vi "save channels to separate multi-tiff files.vi"(8 "frame number in":i32, 9 "last frame":bool, 11 "image data in":dbl[][](array[numeric])) -> ()   [LabVIEW 2012]
doc: "SciScan 1.2 160622"
uses:
  Custom Controls/file format type def.ctl
  GFG/GFGpathGet.vi
  GFG/GFGnumericGet.vi
  GFG/GFGstringGet.vi
  Libtiff3/libtiff3.llb/libtiff3.lvlib
  GFG/GFG library.lvlib
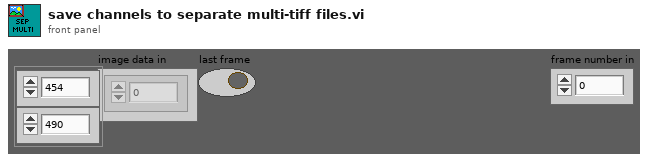
[diagram p1: front panel]
types:
  T1 = typedef "file format type def.ctl" = enum16{"16bit raw", "32bit raw", "16bit multi-tiff (interleave)", "16bit multi-tiff (separate)", "16bit multi-tiff (stacked)", "32bit multi-tiff (interleave)", "32bit multi-tiff (separate)", "32bit multi-tiff (stacked)", "16bit tiff series (interleave)", "16bit tiff series (separate)", "16bit tiff series (stacked)", "32bit tiff series (interleave)", "32bit tiff series (separate)", "32bit tiff series (stacked)"}
  T2 = cluster{"no..of.frames.to.acquire":dbl, "x.pixels":dbl, "y.pixels":dbl, "x.pixel.sz":dbl, "y.pixel.sz":dbl}
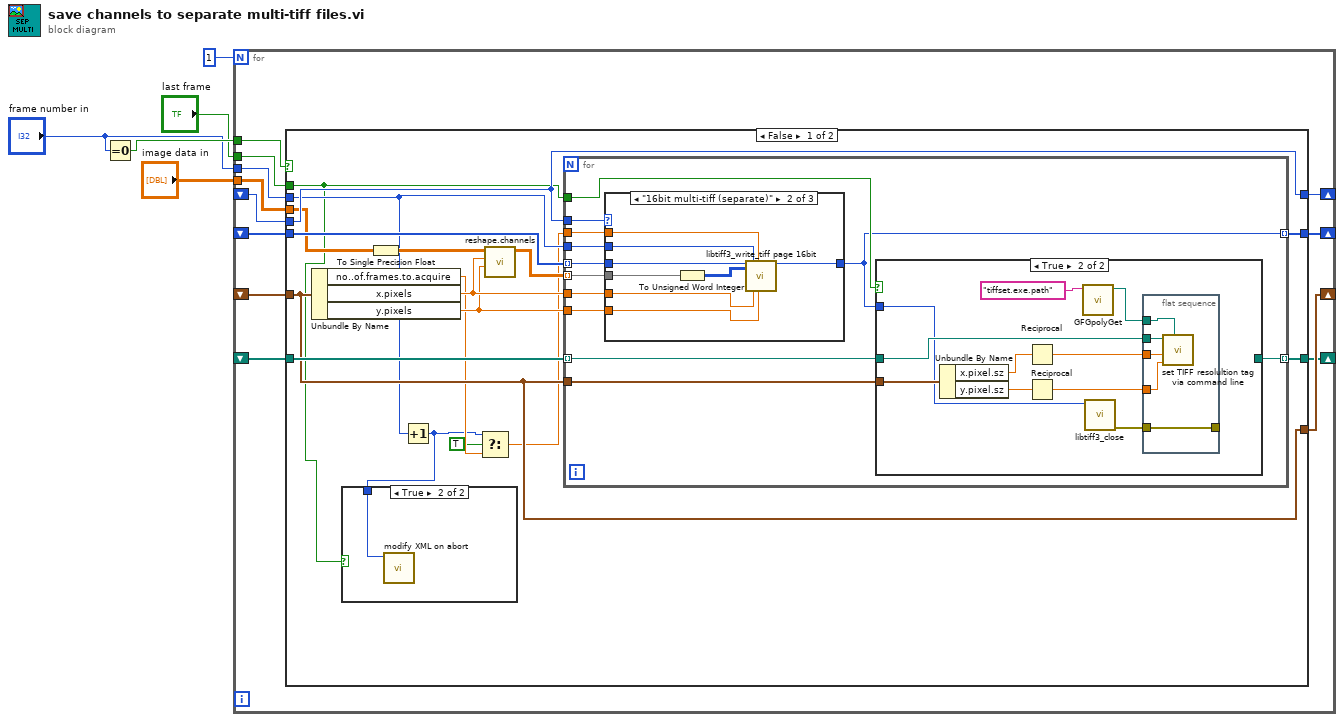
[diagram p0: block diagram]
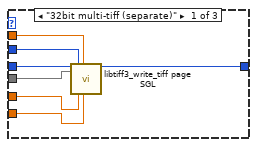
[diagram p3: hidden frame]
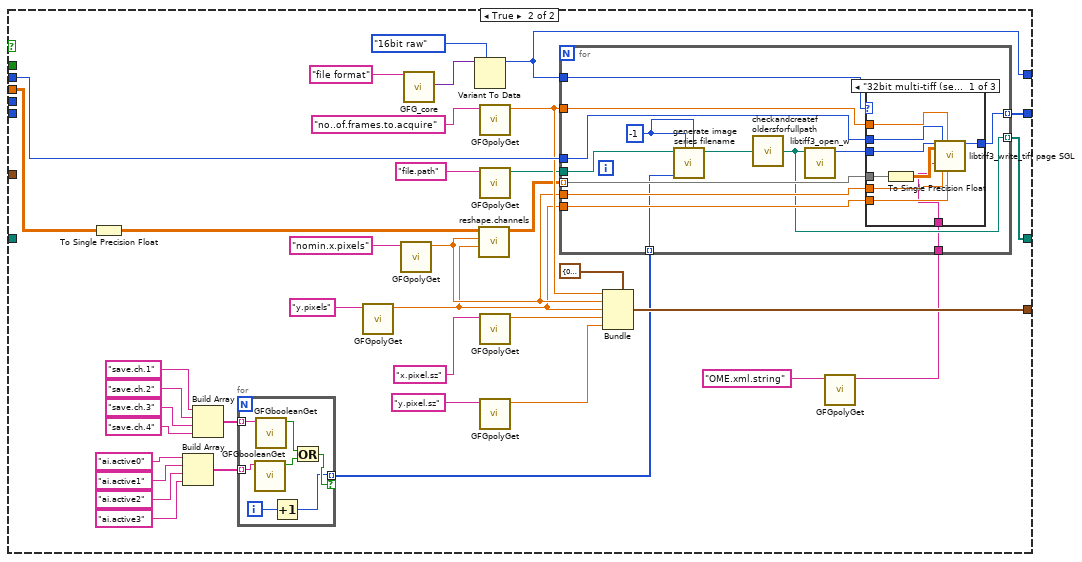
[diagram p6: hidden frame]
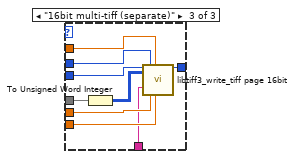
[diagram p8: hidden frame]
diagram:
  n1 = Equal To 0?(x="frame number in") -> (x = 0?=w4:bool)
  n2 = for {
    N: 1 -> [_]
    tunnel: w4 -> [w17]
    shift-right: [w16] -> _
    shift-left: _ -> [w15]
    tunnel: "image data in" -> [w14]
    shift-right: [w13] -> _
    shift-left: _ -> [w12]
    shift-right: [w11] -> _
    shift-left: _ -> [w10]
    shift-right: [w9] -> _
    shift-left: _ -> [w8]
    tunnel: "last frame" -> [w7]
    tunnel: "frame number in" -> [w6]
    n3 = case shown="False" w17 {
      tunnel: w12 -> [w31 _]
      tunnel: [w29 w100] -> w16
      tunnel: w15 -> [w33 _]
      tunnel: w14 -> [w28 w96]
      tunnel: [w31 w103] -> w13
      tunnel: [w30 w104] -> w11
      tunnel: w10 -> [w30 _]
      tunnel: [w32 w93] -> w9
      tunnel: w8 -> [w34 _]
      tunnel: w7 -> [w20 _]
      tunnel: w6 -> [w23 w102]
      frame False {
        n4 = Unbundle By Name(w30) -> ("no..of.frames.to.acquire"=w22:dbl, "x.pixels"=w25:dbl, "y.pixels"=w24:dbl)
        n5 = To Single Precision Float(number=w28) -> (single precision float=w27:sgl[][])
        n6 = Increment(x=w23) -> (x+1=w19:i32)
        n7 = case shown="True" w20 {
          tunnel: w19 -> [_ w35]
          frame False {
          }
          frame True {
            n8 = call "modify XML on abort.vi"("frame number"=w35) -> ()  [unwired: 10 in, 1 out]
          }
        }
        n9 = Select(t=w19, s=TRUE, f=w22) -> (s? t:f=w21:dbl)
        n10 = call "reshape.channels.vi"("y.pixels"=w24, "x.pixels"=w25, "element"=w27) -> ("Array"=w26:dbl[][][])  [unwired: 8 in]
        n11 = for {
          tunnel: w20 -> [w47]
          tunnel: w34 -> [w46] mode=indexing
          tunnel: w26 -> [w45] mode=indexing
          tunnel: w33 -> [w44] mode=indexing
          tunnel: [w43] -> w32 mode=indexing
          tunnel: w21 -> [w42]
          tunnel: w23 -> [w41]
          tunnel: w25 -> [w40]
          tunnel: w24 -> [w39]
          tunnel: w31 -> [w38]
          tunnel: w30 -> [w37]
          tunnel: [w36] -> w29 mode=indexing
          n12 = case shown="\"16bit multi-tiff (separate)\"" w38 {
            tunnel: w45 -> [w48 w62 _]
            tunnel: w44 -> [w54 w60 w63]
            tunnel: [w51 w59 w63] -> w36
            tunnel: w42 -> [w52 w58 _]
            tunnel: w41 -> [w53 w57 _]
            tunnel: w40 -> [w50 w56 _]
            tunnel: w39 -> [w49 w55 _]
            frame "32bit multi-tiff (separate)" {
              n13 = call "libtiff3_write_tiff page SGL.vi"("Handle"=w54, "Image Pixels (Float)"=w48, "page"=w53, "x.pixels"=w50, "totalpages"=w52, "y.pixels"=w49) -> ("Handle out"=w51:i32)  [unwired: 12 in, 1 out]
            }
            frame "16bit multi-tiff (separate)" {
              n14 = To Unsigned Word Integer(number=w62) -> (unsigned 16bit integer=w61:u16[][])
              n15 = call "libtiff3_write_tiff page 16bit.vi"("Handle"=w60, "Image Pixels (U16)"=w61, "page"=w57, "x.pixels"=w56, "totalpages"=w58, "y.pixels"=w55) -> ("Handle out"=w59:i32)  [unwired: 12 in, 1 out]
            }
            frame Default {
            }
          }
          n16 = case shown="True" w47 {
            tunnel: w37 -> [_ w69]
            tunnel: w46 -> [w64 w68]
            tunnel: w36 -> [_ w67]
            tunnel: [w64 _] -> w43
            frame False {
            }
            frame True {
              n17 = Unbundle By Name(w69) -> ("x.pixel.sz"=w70:dbl, "y.pixel.sz"=w71:dbl)
              n18 = Reciprocal(x=w70) -> (1/x=w72:dbl)
              n19 = Reciprocal(x=w71) -> (1/x=w73:dbl)
              n20 = call-poly "GFGpolyGet.vi"("Variable Name in"="tiffset.exe.path") -> ("Path"=w65:path)  [unwired: 8 in, 2 out]
              n21 = call "libtiff3_close.vi"("Handle"=w67) -> ("error out"=w74:errorcluster)  [unwired: 9 in]
              n22 = flat-sequence {
                tunnel: w68 -> [w79]
                tunnel: w74 -> [w76]
                tunnel: w72 -> [w78]
                tunnel: w73 -> [w77]
                tunnel: [w76] -> _
                tunnel: w65 -> [w75]
                frame #0 {
                  n23 = call "set TIFF resolultion tag via command line.vi"("tiffset.exe file path"=w75, "y pixels per m"=w77, "x pixels per m"=w78, "TIFF file path"=w79) -> ()  [unwired: 8 in]
                }
              }
            }
          }
        }
      }
      frame True {
        n24 = To Single Precision Float(number=w96) -> (single precision float=w99:sgl[][])
        n25 = Build Array("ai.active0" ("Variable Name in"), "ai.active1" ("Variable Name in"), "ai.active2" ("Variable Name in"), "ai.active3" ("Variable Name in")) -> (w82:string[])
        n26 = Build Array("save.ch.1" ("Variable Name in"), "save.ch.2" ("Variable Name in"), "save.ch.3" ("Variable Name in"), "save.ch.4" ("Variable Name in")) -> (w87:string[])
        n27 = for {
          tunnel: w87 -> [w123] mode=indexing
          tunnel: w82 -> [w122] mode=indexing
          tunnel: [w117] -> w81 mode=indexing if=w118
          i -> [w119]
          n28 = call "GFGbooleanGet.vi"("Variable Name in"=w122) -> ("Boolean Value OUT"=w121:bool)  [unwired: 9 in, 1 out]
          n29 = call "GFGbooleanGet.vi"("Variable Name in"=w123) -> ("Boolean Value OUT"=w120:bool)  [unwired: 9 in, 1 out]
          n30 = Increment(x=w119) -> (x+1=w117:i32)
          n31 = Or(x=w120, y=w121) -> (x .or. y?=w118:bool)
        }
        n32 = call-poly "GFGpolyGet.vi"("Variable Name in"="y.pixels" ("Tag in")) -> ("Numeric"=w97:dbl)  [unwired: 8 in, 2 out]
        n33 = call-poly "GFGpolyGet.vi"("Variable Name in"="nomin.x.pixels" ("Tag in")) -> ("Numeric"=w98:dbl)  [unwired: 8 in, 2 out]
        n34 = call "GFG_core.vi"("Variable Name in"="file format") -> ("Variant Out"=w115:variant)  [unwired: 12 in, 6 out]
        n35 = Variant To Data(type=file_format_type_def."16bit raw" ("file format"), Variant=w115) -> (data=w103:T1)  [unwired: 1 in, 1 out]
        n36 = call "reshape.channels.vi"("y.pixels"=w97, "x.pixels"=w98, "element"=w99) -> ("Array"=w95:dbl[][][])  [unwired: 8 in]
        n37 = call-poly "GFGpolyGet.vi"("Variable Name in"="no..of.frames.to.acquire") -> ("Numeric"=w101:dbl)  [unwired: 8 in, 2 out]
        n38 = call-poly "GFGpolyGet.vi"("Variable Name in"="file.path") -> ("Path"=w94:path)  [unwired: 8 in, 2 out]
        n39 = call-poly "GFGpolyGet.vi"("Variable Name in"="x.pixel.sz" ("Tag in")) -> ("Numeric"=w107:dbl)  [unwired: 8 in, 2 out]
        n40 = call-poly "GFGpolyGet.vi"("Variable Name in"="y.pixel.sz" ("Tag in")) -> ("Numeric"=w106:dbl)  [unwired: 8 in, 2 out]
        n41 = Bundle(cluster=T2 {"no..of.frames.to.acquire"=0.0, "x.pixels"=0.0, "y.pixels"=0.0, "x.pixel.sz"=0.0, "y.pixel.sz"=0.0} ("output cluster"), "no..of.frames.to.acquire"=w101, "x.pixels"=w98, "y.pixels"=w97, "x.pixel.sz"=w107, "y.pixel.sz"=w106) -> (w104:T2)
        n42 = call-poly "GFGpolyGet.vi"("Variable Name in"="OME.xml.string") -> ("String"=w80:string)  [unwired: 9 in, 1 out]
        n43 = for {
          tunnel: w103 -> [w137]
          tunnel: w102 -> [w136]
          tunnel: w101 -> [w135]
          tunnel: [w134] -> w100 mode=indexing
          tunnel: w98 -> [w133]
          tunnel: w97 -> [w132]
          tunnel: w95 -> [w131] mode=indexing
          tunnel: w94 -> [w129]
          tunnel: [w126] -> w93 mode=indexing
          tunnel: w80 -> [w125]
          tunnel: w81 -> [w124] mode=indexing
          w128 = -1 ("frame number in")
          n44 = call "generate image series filename.vi"("frame number in"=w128, "no..of.frames.to.acquire"=w128, "channel"=w124, "Path IN"=w129) -> ("appended path"=w127:path)  [unwired: 7 in]
          n45 = call "checkandcreatefoldersforfullpath.vi"("Path IN"=w127) -> ("Path OUT"=w126:path)  [unwired: 4 in]
          n46 = call "libtiff3_open_w.vi"("Input path"=w126) -> ("handle"=w130:i32)  [unwired: 9 in, 1 out]
          n47 = case shown="\"32bit multi-tiff (separate)\"" w137 {
            tunnel: w131 -> [w142 _ w153]
            tunnel: w130 -> [w143 w147 w154]
            tunnel: w136 -> [w144 _ w155]
            tunnel: w135 -> [w145 _ w156]
            tunnel: [w146 w147 w149] -> w134
            tunnel: w133 -> [w139 _ w151]
            tunnel: w132 -> [w140 _ w150]
            tunnel: w125 -> [w138 _ w148]
            frame "32bit multi-tiff (separate)" {
              n48 = To Single Precision Float(number=w142) -> (single precision float=w141:sgl[][])
              n49 = call "libtiff3_write_tiff page SGL.vi"("Handle"=w143, "Image Pixels (Float)"=w141, "Image Description"=w138, "page"=w144, "x.pixels"=w139, "totalpages"=w145, "y.pixels"=w140) -> ("Handle out"=w146:i32)  [unwired: 11 in, 1 out]
            }
            frame Default {
            }
            frame "16bit multi-tiff (separate)" {
              n50 = To Unsigned Word Integer(number=w153) -> (unsigned 16bit integer=w152:u16[][])
              n51 = call "libtiff3_write_tiff page 16bit.vi"("Handle"=w154, "Image Pixels (U16)"=w152, "ImageDescription"=w148, "page"=w155, "x.pixels"=w151, "totalpages"=w156, "y.pixels"=w150) -> ("Handle out"=w149:i32)  [unwired: 11 in, 1 out]
            }
          }
        }
      }
    }
  }
